vi "Ecrire dans txt.vi"(0 "Numeric 3":dbl, 1 "Numeric 2":dbl, 2 "Numeric":dbl, 3 "Path":path) -> ()   [LabVIEW 2018]
panel:
  out "String":string
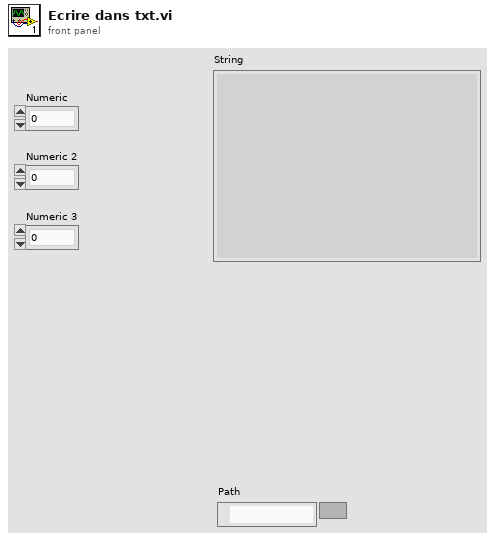
[diagram p1: front panel]
types:
  T1 = enum16{"open", "replace", "create", "open or create", "replace or create", "replace or create with confirmation"}
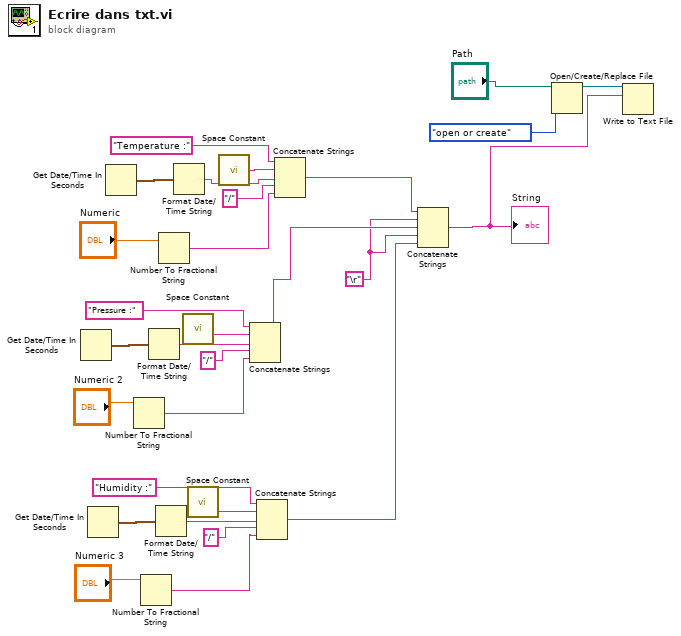
[diagram p0: block diagram]
diagram:
  w9 = "\r"
  n1 = Get Date/Time In Seconds() -> (seconds since 1Jan1904=w26:timestamp)
  n2 = Get Date/Time In Seconds() -> (seconds since 1Jan1904=w23:timestamp)
  n3 = Get Date/Time In Seconds() -> (seconds since 1Jan1904=w29:timestamp)
  n4 = Number To Fractional String(number="Numeric 2") -> (F-format string=w13:string)  [unwired: 3 in]
  n5 = Number To Fractional String(number="Numeric 3") -> (F-format string=w15:string)  [unwired: 3 in]
  n6 = Format Date/Time String(seconds (now)=w26) -> (date/time string=w14:string)  [unwired: 2 in]
  n7 = Format Date/Time String(seconds (now)=w23) -> (date/time string=w17:string)  [unwired: 2 in]
  n8 = Number To Fractional String(number="Numeric") -> (F-format string=w18:string)  [unwired: 3 in]
  n9 = Format Date/Time String(seconds (now)=w29) -> (date/time string=w20:string)  [unwired: 2 in]
  n10 = call <vilib>:"Space Constant.vi"() -> ("String"=w12:string)
  n11 = call <vilib>:"Space Constant.vi"() -> ("String"=w16:string)
  n12 = call <vilib>:"Space Constant.vi"() -> ("String"=w19:string)
  n13 = Concatenate Strings("Pressure :", w12, w14, "/", w13) -> (w10:string)
  n14 = Concatenate Strings("Humidity :", w16, w17, "/", w15) -> (w8:string)
  n15 = Concatenate Strings("Temperature :", w19, w20, "/", w18) -> (w11:string)
  n16 = Concatenate Strings(w11, w9, w10, w9, w8) -> (w1:string)
  "String" <- w1
  n17 = Open/Create/Replace File(file path (use dialog)="Path", operation (0:open)=T1."open or create") -> (refnum out=w2:refnum<file>)  [unwired: 4 in, 2 out]
  n18 = Write to Text File(file (use dialog)=w2, text=w1) -> ()  [unwired: 2 in, 3 out]
